vi "Sample 6 - MoveLoop.vi"() -> ()   [LabVIEW 2016]
panel:
  out "System Index":u32
  in  "Channel":u32
  in  "Position Difference [nm]":i32=8000
  out "Error":errorcluster
  out "State":enum16{"IDLE", "START", "RUN", "STOP"}(ring)
  in  "abort":bool
  out "Exit":bool
  out "connected":bool
  in  "connect":bool
  in  "findSystems":bool caption="Find Systems"
  in  "System locator":string(combo)
  in  "start":bool
  # "A linear positioner with integrated sensor \nshould be connected to channel 0."
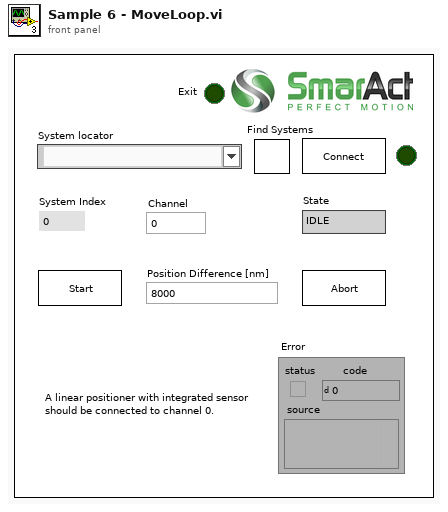
[diagram p1: front panel]
types:
  T1 = enum32{"SA_STOPPED_STATUS", "SA_STEPPING_STATUS", "SA_SCANNING_STATUS", "SA_HOLDING_STATUS", "SA_TARGET_STATUS", "SA_MOVE_DELAY_STATUS", "SA_CALIBRATING_STATUS", "SA_FINDING_REF_STATUS", "SA_OPENING_STATUS"}
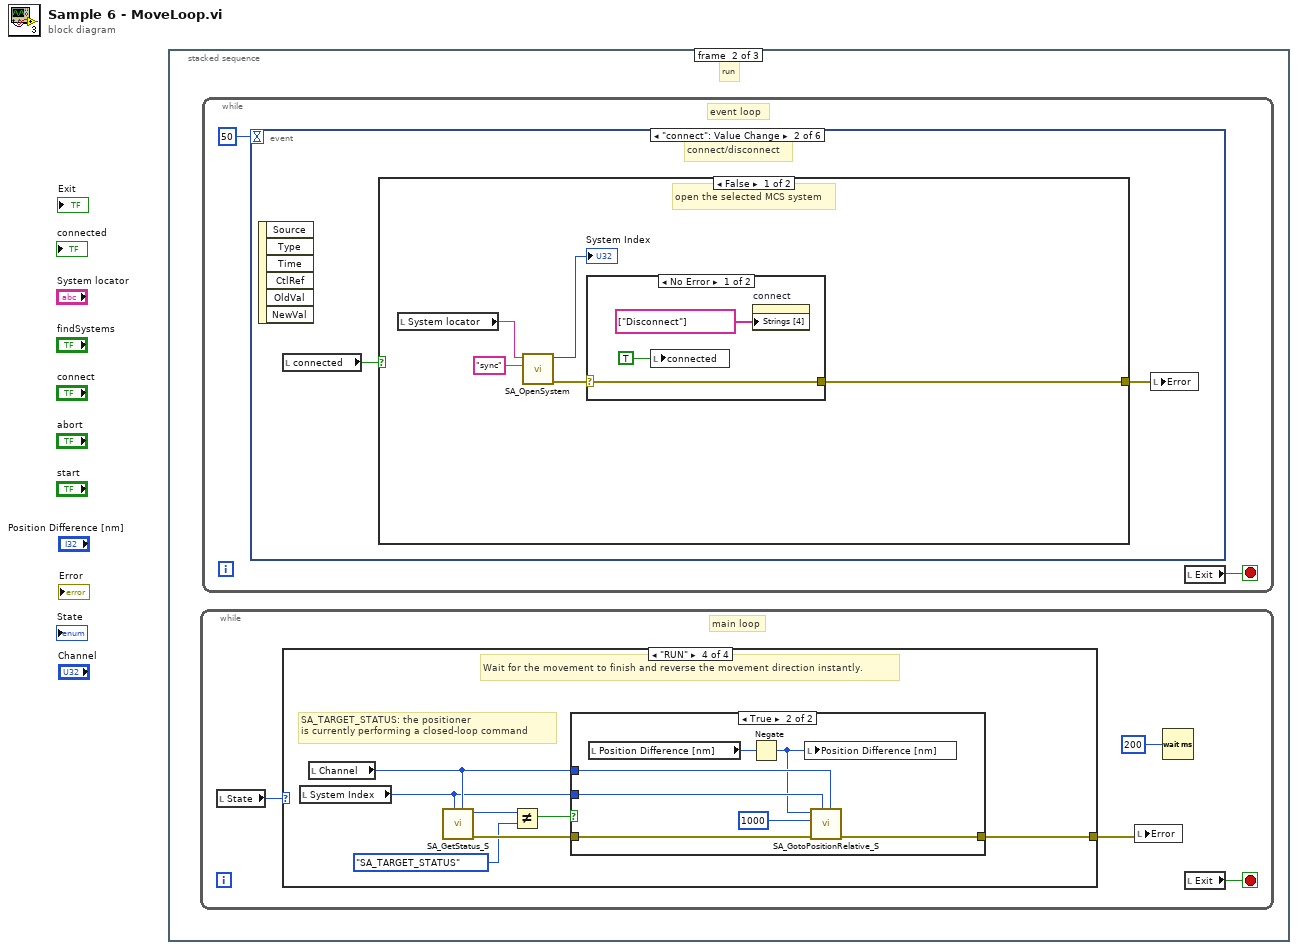
[diagram p0: block diagram]
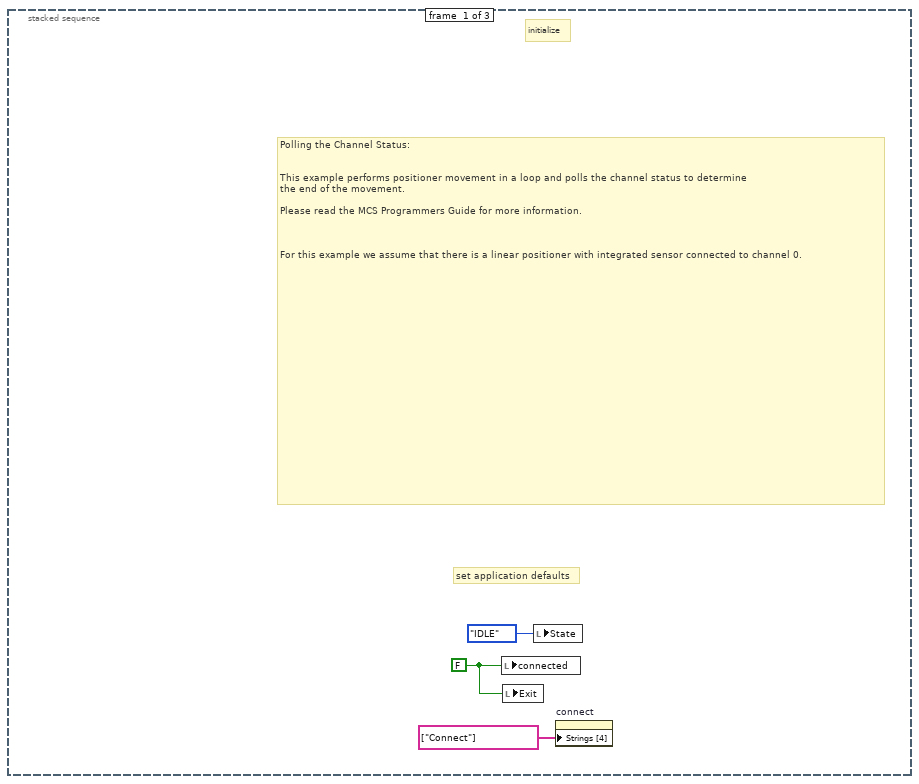
[diagram p2: hidden frame]
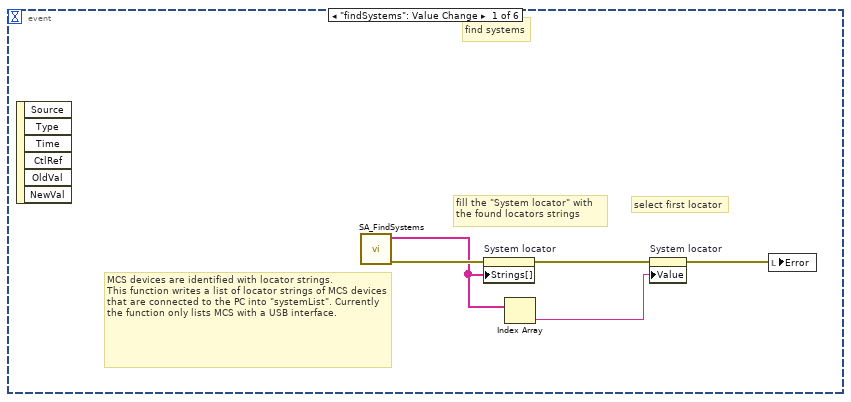
[diagram p3: hidden frame]
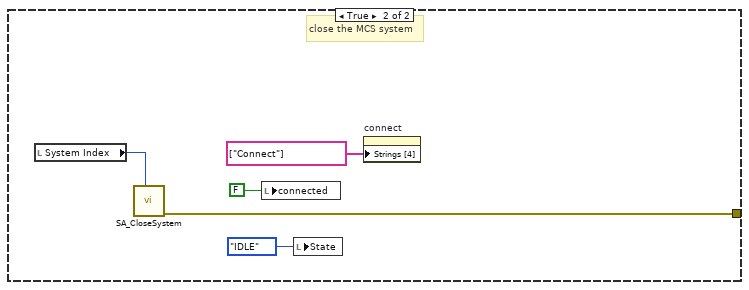
[diagram p5: hidden frame]
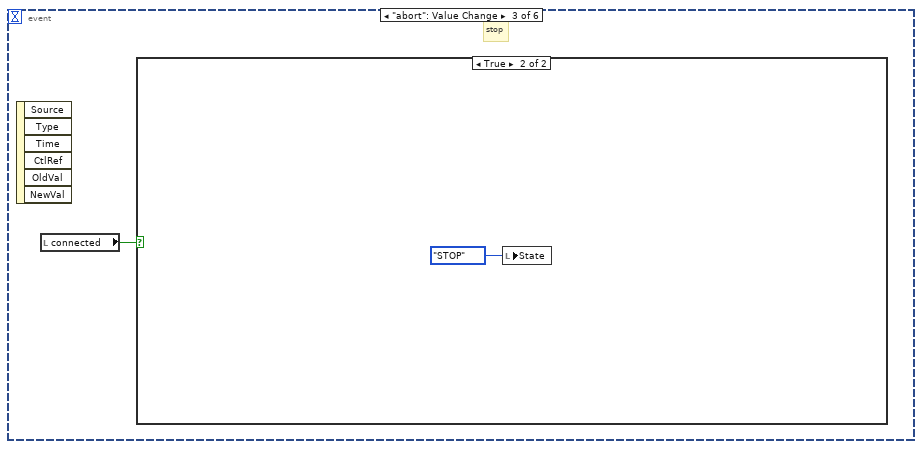
[diagram p6: hidden frame]
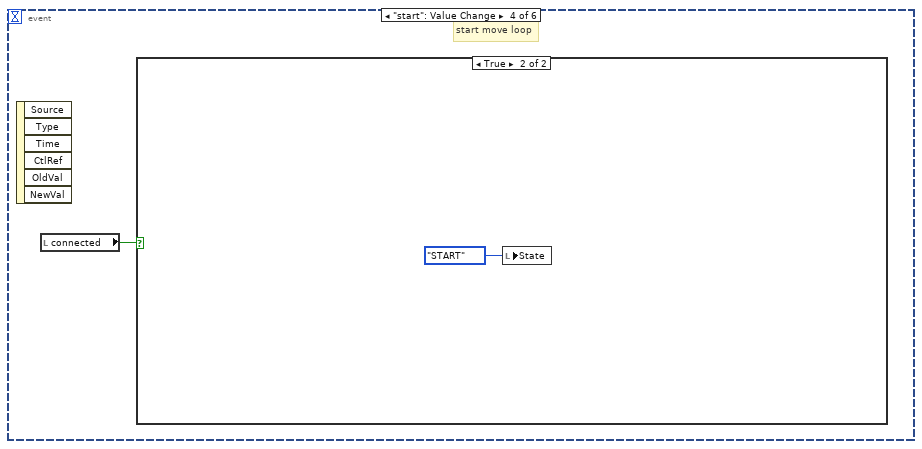
[diagram p8: hidden frame]
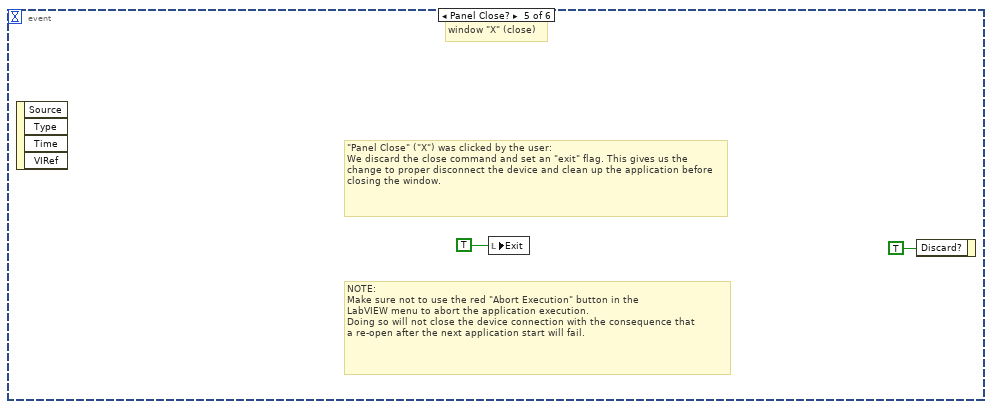
[diagram p10: hidden frame]
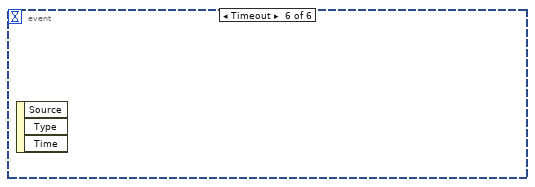
[diagram p11: hidden frame]
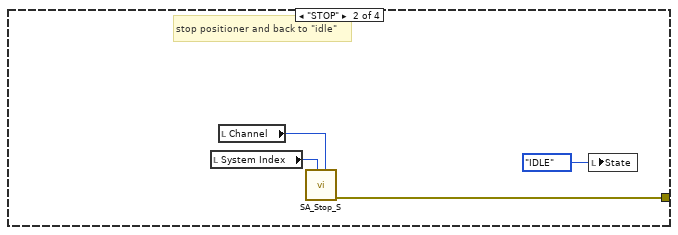
[diagram p13: hidden frame]
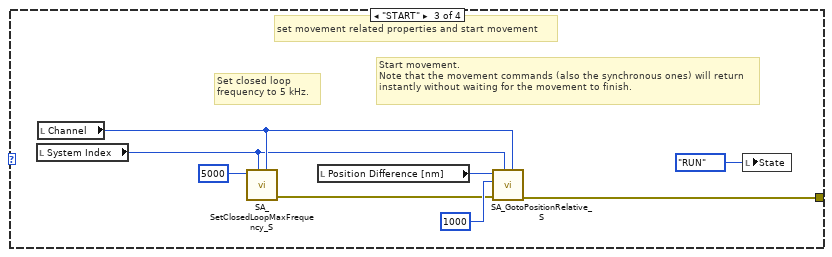
[diagram p14: hidden frame]
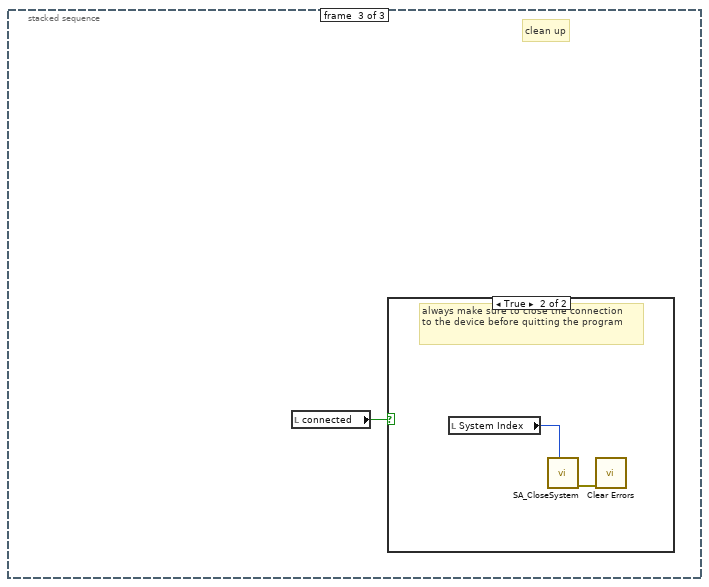
[diagram p16: hidden frame]
diagram:
  n1 = stacked-sequence {
    frame #0 {
      w3 = FALSE ("connected")
      # "Polling the Channel Status:\n\n\nThis example performs positioner movement in a loop and polls the channel status to determine\nthe end of the movement.\n\nPlease read the MCS Programmers Guide for more information.\n\n\n\nFor this example we assume that there is a linear positioner with integrated sensor connected to channel 0."
      # "set application defaults"
      # "initialize"
      n2 = local write "connected"(w3) -> ()
      n3 = local write "Exit"(w3) -> ()
      n4 = local write "State"(enum16{"IDLE", "START", "RUN", "STOP"}."IDLE" ("State")) -> ()
      n5 = property on="connect" class="Bool"("Strings [4]"=string[] ["Connect"]) -> ()  [unwired: 2 in, 2 out]
    }
    frame #1 {
      # "run"
      n6 = while {
        stop <- w36 stop-if-true
        # "main loop"
        n7 = local read "State"() -> (w34:enum16{"IDLE", "START", "RUN", "STOP"})
        n8 = case shown="\"RUN\"" w34 {
          tunnel: [_ w39 w43 w55] -> w33
          frame "IDLE", Default {
            # "nothing to do"
          }
          frame "STOP" {
            # "stop positioner and back to \"idle\""
            n9 = local read "System Index"() -> (w38:u32)
            n10 = local read "Channel"() -> (w37:u32)
            n11 = call <vilib>:"SA_Stop_S.vi"("channelIndex"=w37, "systemIndex"=w38) -> ("error out"=w39:errorcluster)  [unwired: 9 in]
            n12 = local write "State"(enum16{"IDLE", "START", "RUN", "STOP"}."IDLE" ("State")) -> ()
          }
          frame "START" {
            # "Start movement.\nNote that the movement commands (also the synchronous ones) will return instantly without waiting for the movement to finish."
            # "Set closed loop frequency to 5 kHz."
            # "set movement related properties and start movement"
            n13 = local read "System Index"() -> (w41:u32)
            n14 = local read "Channel"() -> (w42:u32)
            n15 = call <vilib>:"SA_SetClosedLoopMaxFrequency_S.vi"("channelIndex"=w42, "systemIndex"=w41, "frequency"=u32 5000 ("MoveVelocity")) -> ("error out"=w44:errorcluster)  [unwired: 8 in]
            n16 = local read "Position Difference [nm]"() -> (w45:i32)
            n17 = call <vilib>:"SA_GotoPositionRelative_S.vi"("channelIndex"=w42, "systemIndex"=w41, "error in (no error)"=w44, "holdTime"=u32 1000 ("MaxCLF"), "diff"=w45) -> ("error out"=w43:errorcluster)  [unwired: 6 in]
            n18 = local write "State"(enum16{"IDLE", "START", "RUN", "STOP"}."RUN" ("State")) -> ()
          }
          frame "RUN" {
            # "SA_TARGET_STATUS: the positioner\nis currently performing a closed-loop command"
            # "Wait for the movement to finish and reverse the movement direction instantly."
            n19 = local read "System Index"() -> (w53:u32)
            n20 = local read "Channel"() -> (w54:u32)
            n21 = call <vilib>:"SA_GetStatus_S.vi"("channelIndex"=w54, "systemIndex"=w53) -> ("error out"=w52:errorcluster, "status"=w50:T1)  [unwired: 8 in]
            n22 = Not Equal?(x=w50, y=T1."SA_TARGET_STATUS") -> (x != y?=w51:bool)
            n23 = case shown="True" w51 {
              tunnel: [w56 w63] -> w55
              tunnel: w52 -> [w56 w62]
              tunnel: w53 -> [_ w61]
              tunnel: w54 -> [_ w60]
              frame False {
              }
              frame True {
                n24 = local read "Position Difference [nm]"() -> (w57:i32)
                n25 = Negate(x=w57) -> (-x=w59:i32)
                n26 = local write "Position Difference [nm]"(w59) -> ()
                n27 = call <vilib>:"SA_GotoPositionRelative_S.vi"("channelIndex"=w60, "systemIndex"=w61, "error in (no error)"=w62, "holdTime"=u32 1000, "diff"=w59) -> ("error out"=w63:errorcluster)  [unwired: 6 in]
              }
            }
          }
        }
        n28 = local write "Error"(w33) -> ()
        n29 = Wait (ms)(milliseconds to wait=u32 200) -> ()  [unwired: 1 out]
        n30 = local read "Exit"() -> (w36:bool)
      }
      n31 = while {
        stop <- w4 stop-if-true
        # "event loop"
        n32 = event shown="[1] \"connect\": Value Change" {
          selector: _ -> [_ _ _ _ _ _]
          dyn-events: _ -> [_ _ _ _ _ _]
          timeout: 50 -> [_ _ _ _ _ _]
          event "findSystems": Value Change {
            # "select first locator"
            # "fill the \"System locator\" with\nthe found locators strings"
            # "MCS devices are identified with locator strings.\nThis function writes a list of locator strings of MCS devices that are connected to the PC into \"systemList\". Currently the function only lists MCS with a USB interface."
            # "find systems"
            n33 = event-data() -> ()  [unwired: 1 in, 6 out]
            n34 = call <vilib>:"SA_FindSystems.vi"() -> ("error out"=w10:errorcluster, "systemList"=w9:string[])  [unwired: 10 in]
            n35 = property on="System locator" class="CmbBox"(error in=w10, "Strings[]"=w9) -> (error out=w8:errorcluster)  [unwired: 1 in, 1 out]
            n36 = Index Array(array=w9) -> (element=w7:string)  [unwired: 1 in]
            n37 = property on="System locator" class="CmbBox"(error in=w8, "Value"=w7) -> (error out=w6:errorcluster)  [unwired: 1 in, 1 out]
            n38 = local write "Error"(w6) -> ()
          }
          event "connect": Value Change {
            # "connect/disconnect"
            n39 = event-data() -> ()  [unwired: 1 in, 6 out]
            n40 = local read "connected"() -> (w12:bool)
            n41 = case shown="False" w12 {
              tunnel: [w15 w23] -> w11
              frame False {
                # "open the selected MCS system"
                n42 = local read "System locator"() -> (w16:string)
                n43 = call <vilib>:"SA_OpenSystem.vi"("options"="sync", "systemLocator"=w16) -> ("error out"=w17:errorcluster, "systemIndexOut"=→"System Index":u32)  [unwired: 8 in]
                n44 = case shown="No Error" w17 {
                  selector: w17 -> [w18 w21]
                  tunnel: [w18 w21] -> w15
                  frame No Error {
                    n45 = local write "connected"(TRUE ("connected")) -> ()
                    n46 = property on="connect" class="Bool"("Strings [4]"=string[] ["Disconnect"]) -> ()  [unwired: 2 in, 2 out]
                  }
                  frame Error {
                  }
                }
              }
              frame True {
                # "close the MCS system"
                n47 = local read "System Index"() -> (w26:u32)
                n48 = call <vilib>:"SA_CloseSystem.vi"("systemIndex"=w26) -> ("error out"=w23:errorcluster)  [unwired: 10 in]
                n49 = local write "connected"(FALSE ("connected")) -> ()
                n50 = local write "State"(enum16{"IDLE", "START", "RUN", "STOP"}."IDLE" ("State")) -> ()
                n51 = property on="connect" class="Bool"("Strings [4]"=string[] ["Connect"]) -> ()  [unwired: 2 in, 2 out]
              }
            }
            n52 = local write "Error"(w11) -> ()
          }
          event "abort": Value Change {
            # "stop"
            n53 = event-data() -> ()  [unwired: 1 in, 6 out]
            n54 = local read "connected"() -> (w27:bool)
            n55 = case shown="True" w27 {
              frame False {
              }
              frame True {
                n56 = local write "State"(enum16{"IDLE", "START", "RUN", "STOP"}."STOP" ("State")) -> ()
              }
            }
          }
          event "start": Value Change {
            # "start move loop"
            n57 = event-data() -> ()  [unwired: 1 in, 6 out]
            n58 = local read "connected"() -> (w29:bool)
            n59 = case shown="True" w29 {
              frame False {
              }
              frame True {
                n60 = local write "State"(enum16{"IDLE", "START", "RUN", "STOP"}."START" ("State")) -> ()
              }
            }
          }
          event Panel Close? {
            # "NOTE:\nMake sure not to use the red \"Abort Execution\" button in the\nLabVIEW menu to abort the application execution.\nDoing so will not close the device connection with the consequence that\na re-open after the next application start will fail."
            # "\"Panel Close\" (\"X\") was clicked by the user:\nWe discard the close command and set an \"exit\" flag. This gives us the change to proper disconnect the device and clean up the application before closing the window."
            # "window \"X\" (close)"
            n61 = event-data() -> ()  [unwired: 1 in, 4 out]
            n62 = local write "Exit"(TRUE ("exit")) -> ()
            n63 = event-data("Discard?"=TRUE) -> ()  [unwired: 1 in, 1 out]
          }
          event Timeout {
            n64 = event-data() -> ()  [unwired: 1 in, 3 out]
          }
        }
        n65 = local read "Exit"() -> (w4:bool)
      }
    }
    frame #2 {
      # "clean up"
      n66 = local read "connected"() -> (w64:bool)
      n67 = case shown="True" w64 {
        frame False {
        }
        frame True {
          # "always make sure to close the connection\nto the device before quitting the program"
          n68 = local read "System Index"() -> (w66:u32)
          n69 = call <vilib>:"SA_CloseSystem.vi"("systemIndex"=w66) -> ("error out"=w65:errorcluster)  [unwired: 10 in]
          n70 = call <vilib>:"Clear Errors.vi"("error in (no error)"=w65) -> ()  [unwired: 5 in, 2 out]
        }
      }
    }
  }
